vi "PID-FM.vi"() -> ()   [LabVIEW 2012]
panel:
  out "Numeric":dbl
  in  "Phase (Degree) Shift":dbl
  in  "PID Stop":bool
  out "PID Input Error":dbl
  in  "Proportional Gain":ext
  in  "Integral Gain":dbl
  out "P+I Error":dbl
  out "Phase (Rad) Shift Difference":dbl
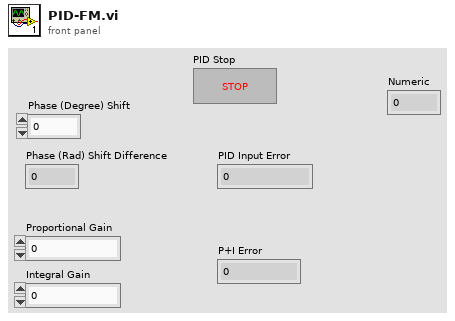
[diagram p1: front panel]
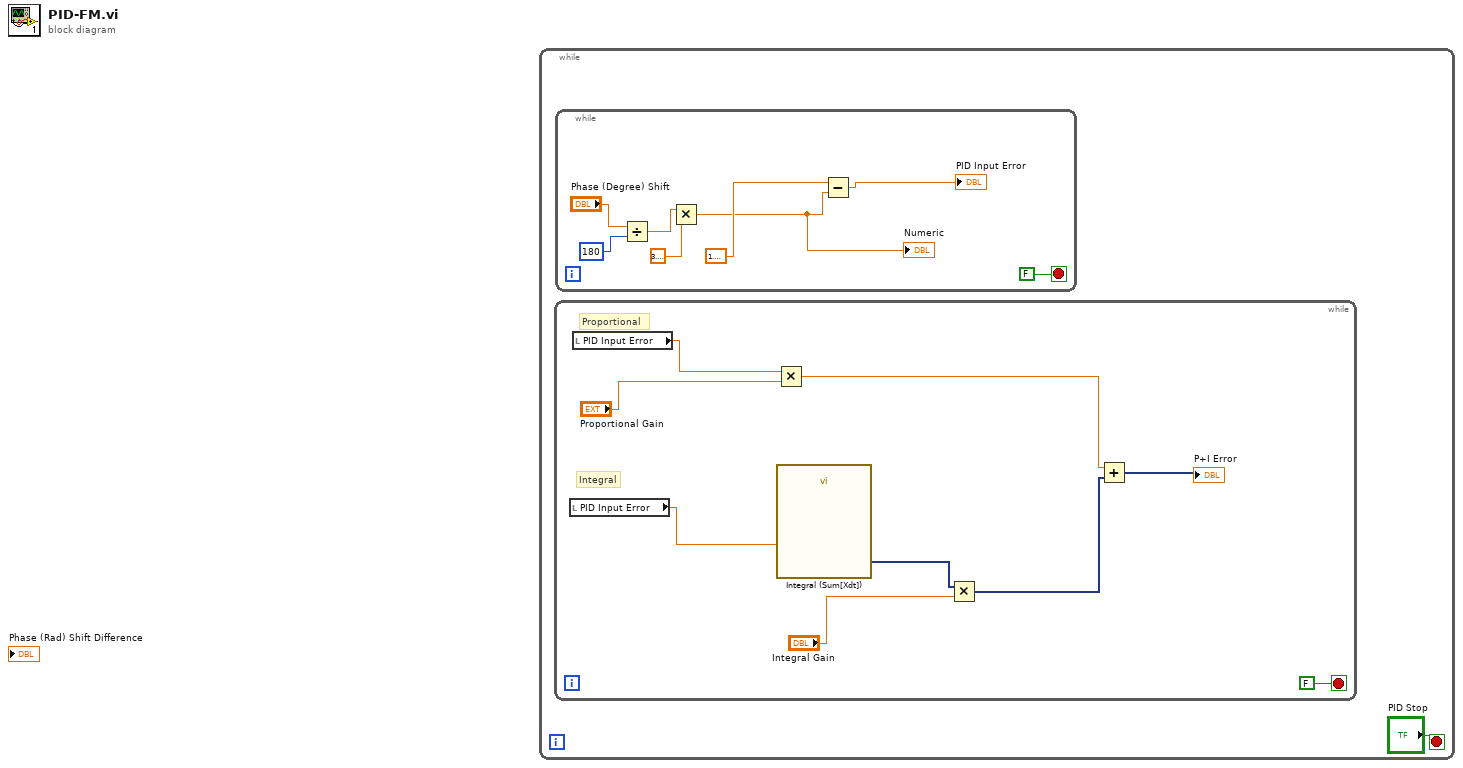
[diagram p0: block diagram]
diagram:
  n1 = while {
    stop <- "PID Stop" stop-if-true
    n2 = while {
      stop <- FALSE stop-if-true
      # "Integral"
      # "Proportional"
      n3 = local read "PID Input Error"() -> (w15:dbl)
      n4 = local read "PID Input Error"() -> (w17:dbl)
      n5 = Multiply(x=w17, y="Proportional Gain") -> (x*y=w12:ext)
      n6 = call "Integral (Sum[Xdt])"("Signals"=w15) -> ("Result"=w14:dynamicdata)  [unwired: 5 in, 1 out]
      n7 = Multiply(x=w14, y="Integral Gain") -> (x*y=w11:dynamicdata)
      n8 = Add(x=w12, y=w11) -> (x+y=→"P+I Error":dynamicdata)
    }
    n9 = while {
      stop <- FALSE stop-if-true
      n10 = Divide(x="Phase (Degree) Shift", y=180) -> (x/y=w5:dbl)
      n11 = Multiply(x=w5, y=3.141592653589793) -> (x*y=w3:dbl)
      "Numeric" <- w3
      n12 = Subtract(x=1.5707963267948966, y=w3) -> (x-y=→"PID Input Error":dbl)
    }
  }
